vi "dvp Vi Get Sharpness.vi"(10 "pSharpness":i32, 11 "handle":u32) -> (2 "pSharpness out":i32, 3 "function return":u32(ring))   [LabVIEW 2018, in "LabViewDVPCamera.lvlib"]
doc: "LabviewDvp2Api dvpStatus dvpViGetSharpness(dvpHandle handle, dvpInt32 *pSharpness);"
uses:
  LabViewDVPCamera.lvlib
  LabViewDVPCamera/LabViewDVPCamera.dll
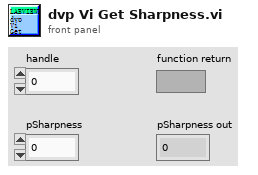
[diagram p1: front panel]
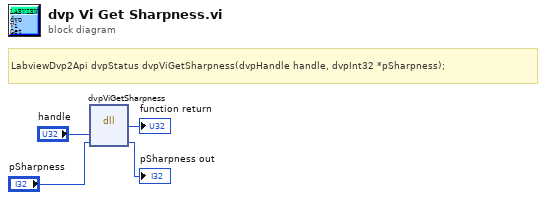
[diagram p0: block diagram]
diagram:
  # "LabviewDvp2Api dvpStatus dvpViGetSharpness(dvpHandle handle, dvpInt32 *pSharpness);"
  n1 = dll-call lib="C:/Program Files (x86)/DVP2 Labview cn 64/Sample/LabViewDVPCamera/LabViewDVPCamera.*" fn="dvpViGetSharpness"("handle"="handle", "pSharpness"="pSharpness") -> (→"function return":u32, "pSharpness"=→"pSharpness out":i32)  [unwired: 4 in, 2 out]
